vi "Scan1762WithPumpingHWT.vi"() -> ()   [LabVIEW 2012]
uses:
  <vilib>/Utility/file.llb/Write To Spreadsheet File (DBL).vi
panel:
  in  "Comment":string="SPAOM, 3000 mA, 60 mA, 150 mA, now being mixed with 20 MHz, 7V Res, 89 MHz DPAOM"
  in  "B Field":dbl=3.0
  in  "Power":dbl=4.0
  in  "Runs per data point":dbl=100.0
  in  "Step Size":dbl(slide)=2000.0 min=100.0 max=100000.0 step=1.0 scale=100.0..100000.0 scale format="%#.0f"
  in  "Low Freq":dbl(slide)=78950000.0 min=50000000.0 max=120000000.0 step=1000.0 scale=50000000.0..120000000.0 scale format="%#.5f"
  in  "High Freq":dbl(slide)=79060000.0 min=50000000.0 max=120000000.0 step=1000.0 scale=50000000.0..120000000.0 scale format="%#.0f"
  out "Cur Freq":dbl=78998000.0 format="%#_8f"
  out "Path":path=path "c:/data/1762 Scans/2009-11-09_16-22-05_1762scanWithPumping.txt"
  out "Frequency Scan":cluster{dbl, dbl}[](graph)=[{79100000.0, 0.0}, {79098000.0, 0.01}, {79096000.0, 0.0}, {79094000.0, 0.0}, {79092000.0, 0.0}, {79090000.0, 0.01}, {79088000.0, 0.0}, {79086000.0, 0.0}, {79084000.0, 0.0}, {79082000.0, 0.0}, {79080000.0, 0.0}, {79078000.0, 0.0}, {79076000.0, 0.0}, {79074000.0, 0.02}, {79072000.0, 0.0}, {79070000.0, 0.0}, {79068000.0, 0.0}, {79066000.0, 0.0}, {79064000.0, 0.01}, {79062000.0, 0.0}, {79060000.0, 0.0}, {79058000.0, 0.02}, {79056000.0, 0.01}, {79054000.0, 0.01}, {79052000.0, 0.02}, {79050000.0, 0.01}, {79048000.0, 0.01}, {79046000.0, 0.05}, {79044000.0, 0.01}, {79042000.0, 0.01}, {79040000.0, 0.04}, {79038000.0, 0.02}, {79036000.0, 0.07}, {79034000.0, 0.07}, {79032000.0, 0.04}, {79030000.0, 0.08}, {79028000.0, 0.16}, {79026000.0, 0.22}, {79024000.0, 0.27}, {79022000.0, 0.31}, {79020000.0, 0.37}, {79018000.0, 0.49}, {79016000.0, 0.44}, {79014000.0, 0.36}, {79012000.0, 0.37}, {79010000.0, 0.48}, {79008000.0, 0.23}, {79006000.0, 0.29}, {79004000.0, 0.02}, {79002000.0, 0.02}, {79000000.0, 0.11}]
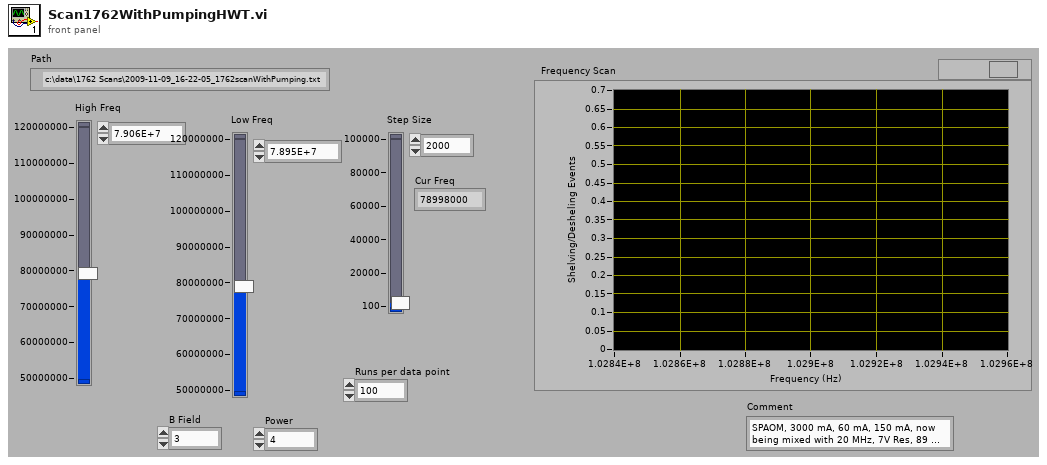
[diagram p1: front panel]
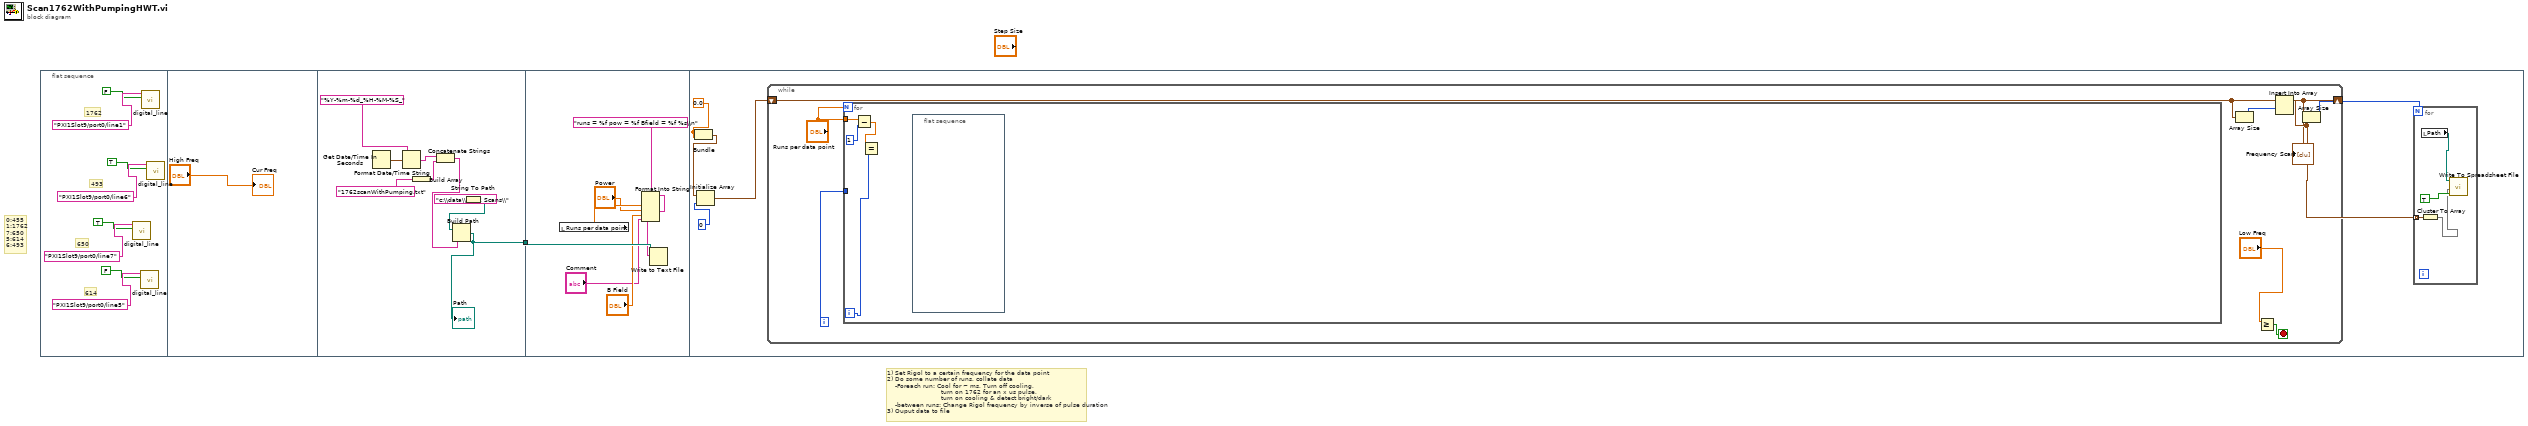
[diagram p0: block diagram]
diagram:
  # "1) Set Rigol to a certain frequency for the data point\n2) Do some number of runs, collate data\n    -Foreach run: Cool for ~ ms, Turn off cooling,\n                           turn on 1762 for an x us pulse,\n                           turn on cooling & detect bright/dark\n    -between runs: Change Rigol frequency by inverse of pulse duration\n3) Ouput data to file"
  # "0:455\n1:1762\n7:650\n5:614\n6:493"
  n1 = flat-sequence {
    tunnel: [w11] -> w1
    tunnel: w1 -> [w26]
    frame #0 {
      # "614"
      # "650"
      # "493"
      # "1762"
      n2 = call "digital_line.vi"("Boolean"=TRUE, "lines"=tag "PXI1Slot9/port0/line7") -> ()  [unwired: 5 in, 1 out]
      n3 = call "digital_line.vi"("Boolean"=FALSE, "lines"=tag "PXI1Slot9/port0/line5") -> ()  [unwired: 5 in, 1 out]
      n4 = call "digital_line.vi"("Boolean"=FALSE, "lines"=tag "PXI1Slot9/port0/line1") -> ()  [unwired: 5 in, 1 out]
      n5 = call "digital_line.vi"("Boolean"=TRUE, "lines"=tag "PXI1Slot9/port0/line6") -> ()  [unwired: 5 in, 1 out]
    }
    frame #1 {
      "Cur Freq" <- "High Freq"
    }
    frame #2 {
      n6 = Get Date/Time In Seconds() -> (seconds since 1Jan1904=w13:timestamp)
      n7 = Format Date/Time String(time format string (%c)="%Y-%m-%d_%H-%M-%S_", seconds (now)=w13) -> (date/time string=w15:string)  [unwired: 1 in]
      n8 = Build Array("1762scanWithPumping.txt") -> (w18:string[])
      n9 = Concatenate Strings(w15, w18) -> (w17:string)
      n10 = String To Path(string="c:\\data\\1762 Scans\\") -> (path=w19:path)
      n11 = Build Path(base path=w19, name or relative path=w17) -> (appended path=w11:path)
      "Path" <- w11
    }
    frame #3 {
      n12 = local read "Runs per data point"() -> (w23:dbl)
      n13 = Format Into String(format string="runs = %f pow = %f Bfield = %f %s\\n", w23, "Power", "B Field", "Comment") -> (resulting string=w24:string)  [unwired: 2 in, 1 out]
      n14 = Write to Text File(file (use dialog)=w26, text=w24) -> ()  [unwired: 2 in, 3 out]
    }
    frame #4 {
      w31 = 0.0
      n15 = Bundle(w31, w31) -> (w32:cluster{dbl, dbl})  [unwired: 1 in]
      n16 = Initialize Array(w32, 0) -> (w29:cluster{dbl, dbl}[])
      n17 = while {
        shift-right: [w38] -> w27
        shift-left: w29 -> [w39]
        i -> [w43]
        stop <- w41 stop-if-true
        n18 = for {
          N: "Runs per data point" -> [_]
          tunnel: w43 -> [_]
          tunnel: "Runs per data point" -> [w45]
          i -> [w44]
          n19 = Subtract(x=w45, y=1) -> (x-y=w47:dbl)
          n20 = Equal?(x=w47, y=w44) -> ()  [unwired: 1 out]
          n21 = flat-sequence {
            frame #0 {
            }
          }
        }
        n22 = Array Size(array=w39) -> (size(s)=w40:i32)
        n23 = Greater Or Equal?(x="Low Freq") -> (x >= y?=w41:bool)  [unwired: 1 in]
        n24 = Insert Into Array(array=w39, index=w40) -> (w38:cluster{dbl, dbl}[])  [unwired: 1 in]
        "Frequency Scan" <- w38
      }
      n25 = Array Size(array=w27) -> (size(s)=w28:i32)
      n26 = for {
        N: w28 -> [_]
        tunnel: w27 -> [w36] mode=indexing
        n27 = local read "Path"() -> (w33:path)
        n28 = Cluster To Array(cluster=w36) -> (array=w34:dbl[])
        n29 = call-poly <vilib>:"Write To Spreadsheet File.vi"("append to file? (new file:F)"=TRUE, "1D data"=w34, "file path (dialog if empty)"=w33) -> ()  [unwired: 5 in, 1 out]
      }
    }
  }
